vi "DataSocket-ImageReader.vi"() -> ()   [LabVIEW 2019]
doc: "Uses DataSocket to read array data. \n \nThe Writer, Server, and Reader can all be on the same computer or different computers. The Writer and Reader URLs should point to the computer where the DataSocket Server is."
uses:
  <vilib>/vision/Image Controls.llb/IMAQ Image.ctl
panel:
  out "Image":T1(plugin-control)
  in  "Stop":bool
  # "DataSocket - Image Receiver"
  # "Instruction:\n1. Run DataSocket Server;\n2. Run Image Receiver.\n3. Run this VI;\n4. See the images received\n     from Sender."
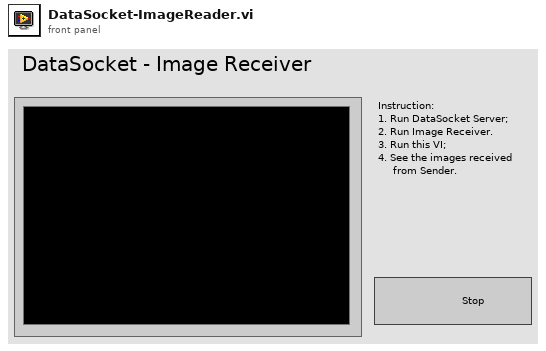
[diagram p1: front panel]
types:
  T1 = typedef "IMAQ Image.ctl" = refnum<image>
  T2 = enum16{"Read", "Write", "ReadWrite", "BufferedRead", "BufferedReadWrite"}
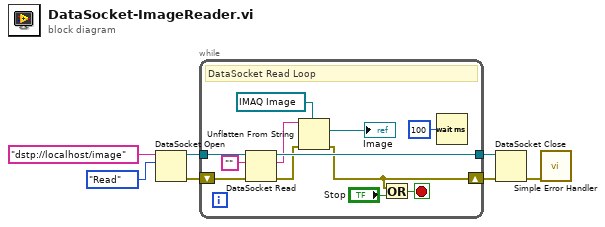
[diagram p0: block diagram]
diagram:
  n1 = DataSocket Open(10:T2."Read" ("mode"), 11:"dstp://localhost/image" ("Read Location")) -> (0:w5:errorcluster, 3:w6:refnum<k13>)  [unwired: 2 in]
  n2 = while {
    tunnel: w6 -> [w17]
    tunnel: [w15] -> w1
    shift-right: [w10] -> w4
    shift-left: w5 -> [w16]
    stop <- w18 stop-if-true
    # "DataSocket Read Loop"
    n3 = DataSocket Read(8:w16, 10:"", 11:w17) -> (0:w11:errorcluster, 2:w13:string, 3:w15:refnum<k13>)  [unwired: 1 in, 5 out]
    n4 = Unflatten From String(type=T1 refnum ("Image"), binary string=w13, error in (no error)=w11) -> (value=→"Image":T1, error out=w10:errorcluster)  [unwired: 2 in, 1 out]
    n5 = Or(x=w10, y="Stop") -> (x .or. y?=w18:bool)
    n6 = Wait (ms)(milliseconds to wait=u32 100) -> ()  [unwired: 1 out]
  }
  n7 = DataSocket Close(8:w4, 11:w1) -> (0:w2:errorcluster)  [unwired: 1 in, 1 out]
  n8 = call <vilib>:"Simple Error Handler.vi"("error in (no error)"=w2) -> ()  [unwired: 4 in, 5 out]
